vi "CODMn测量流程.vi"(11 "控制命令":u16(ring)=1 items=["启动测量"=1, "标样核查"=2, "零点核查"=3, "跨度核查"=4, "空白测试"=5, "平行样测试"=6, "加标回收"=7, "空白校准"=8, "标样校准"=9, "初始化（清洗）"=10, "停止测试"=11, "仪器重启"=12, "校时"=13, "模式设置"=14, "测量间隔设置"=15, "调试"=22, "填充管路"=30, "清洗管路"=31, "清洗反应杯"=32]) -> ()   [LabVIEW 2016, in "斯坦道CODMn新电路板.lvlib"]
panel:
  out "start":timestamp
  out "补测":bool
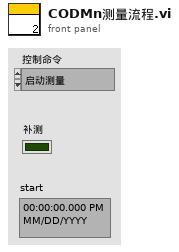
[diagram p1: front panel]
types:
  T1 = cluster{"时间标识":timestamp, "设备":string, "日志信息":string, "流程参数":string}
  T2 = cluster{"站号":u16, "量程切换":enum32{"H", "L", "AUTO"}, "控制命令":u16, "模式设置":enum16{"待机", "连续模式", "周期模式", "定点模式", "受控模式", "手动模式"}, "测量间隔":u16}
  T3 = cluster{"系统时间":timestamp, "工作状态":u16, "测量模式":enum16{"待机", "连续模式", "周期模式", "定点模式", "受控模式", "手动模式"}, "告警代码":u16, "故障代码":u16, "日志代码":u16, "软件版本":u16, "A":sgl, "B":sgl, "K":sgl, "当前滴定数":sgl, "T":sgl, "H":sgl, "id":u16, "flowid":u16, "量程":u16, "加热实时温度":sgl, "当前ORP值":sgl, "运行时间":sgl, "当前步骤剩余时间":sgl, "结束滴定数":sgl, "注射泵保温温度":sgl, "匹配滴定数X0":u16, "X^2":sgl, "X":sgl, "B 2":sgl, "光值1":sgl, "光值2":sgl, "光值3":sgl, "光值4":sgl, "光值5":sgl, "光值6":sgl, "光值7":sgl, "光值8":sgl}
  T4 = cluster{"因子编码":u32, "单位":u16, "标样参考值":sgl, "水样数据时间":timestamp, "水样实测值":sgl, "水样数据标识":string, "标样数据时间":timestamp, "标样实测值":sgl, "标样数据标识":string, "空白数据时间":timestamp, "空白实测值":sgl, "空白数据标识":string, "零点核查数据时间":timestamp, "零点核查实测值":sgl, "零点核查数据标识":string, "跨度核查数据时间":timestamp, "跨度核查实测值":sgl, "跨度核查数据标识":string, "加标回收数据时间":timestamp, "加标回收实测值":sgl, "加标回收数据标识":string, "平行样数据时间":timestamp, "平行样实测值":sgl, "平行样数据标识":string, "F0":sgl, "F1":sgl, "F2":sgl, "F3":sgl, "F4":sgl, "F5":sgl, "F6":sgl, "F7":sgl, "温度":sgl, "湿度":sgl, "X值":sgl, "fidrange":u16}
  T5 = cluster{"跨度值":dbl, "零点标准液浓度":dbl, "跨度标准液浓度":dbl, "标准液标准浓度":dbl, "零点标准液偏差":dbl, "跨度标准液偏差":dbl, "标准液标准偏差":dbl}
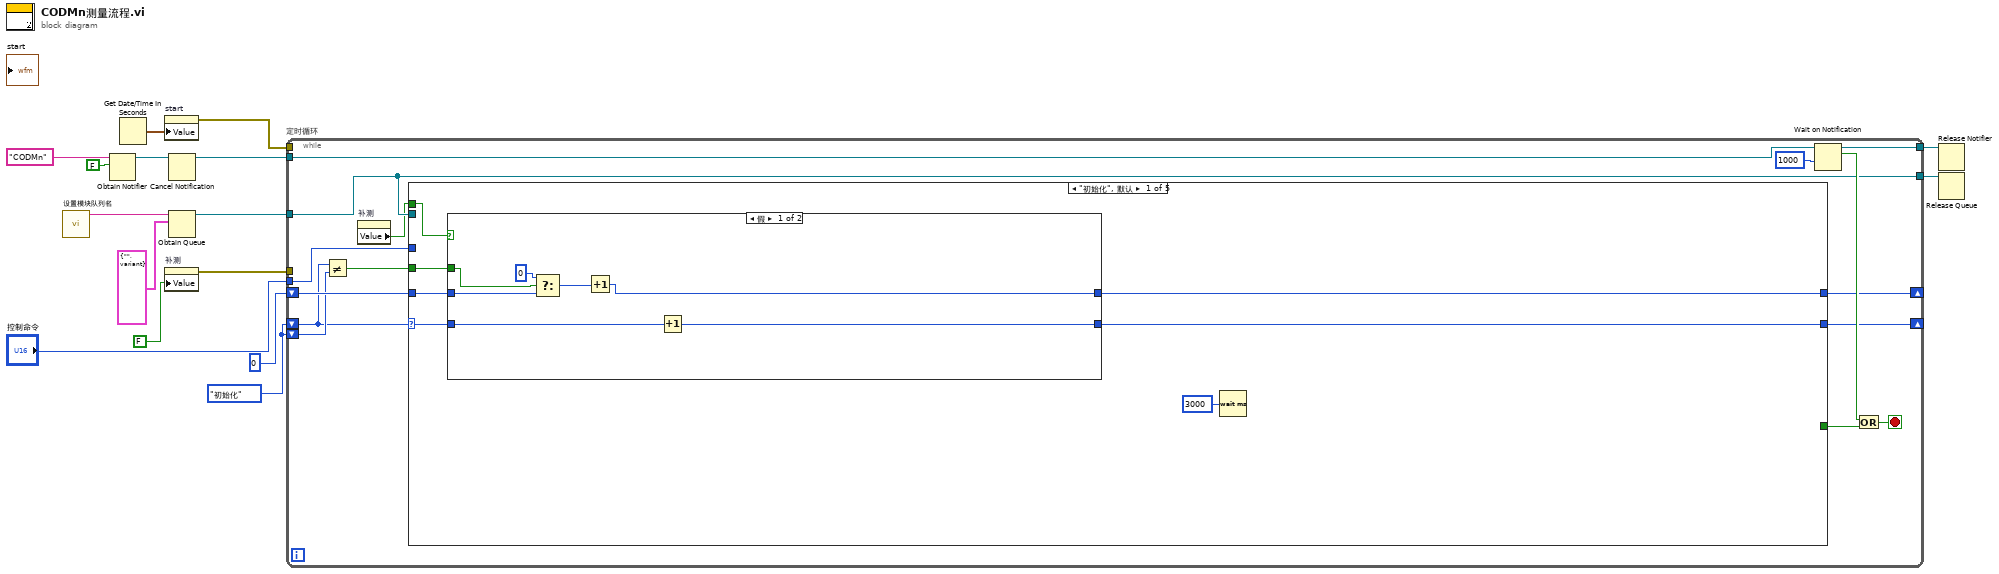
[diagram p0: block diagram]
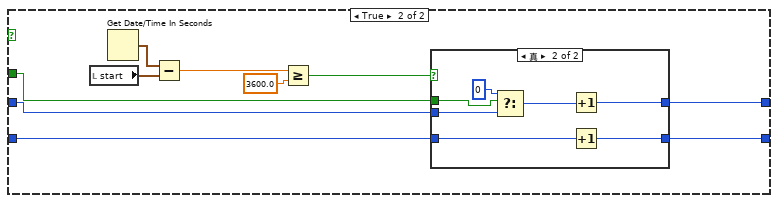
[diagram p2: hidden frame]
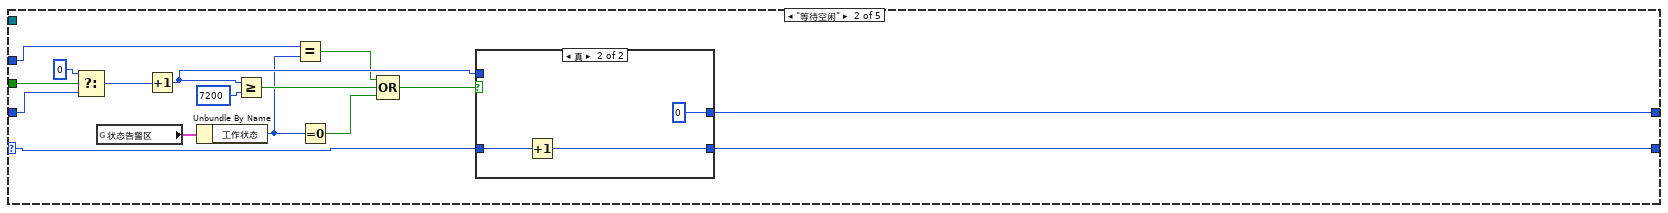
[diagram p4: hidden frame]
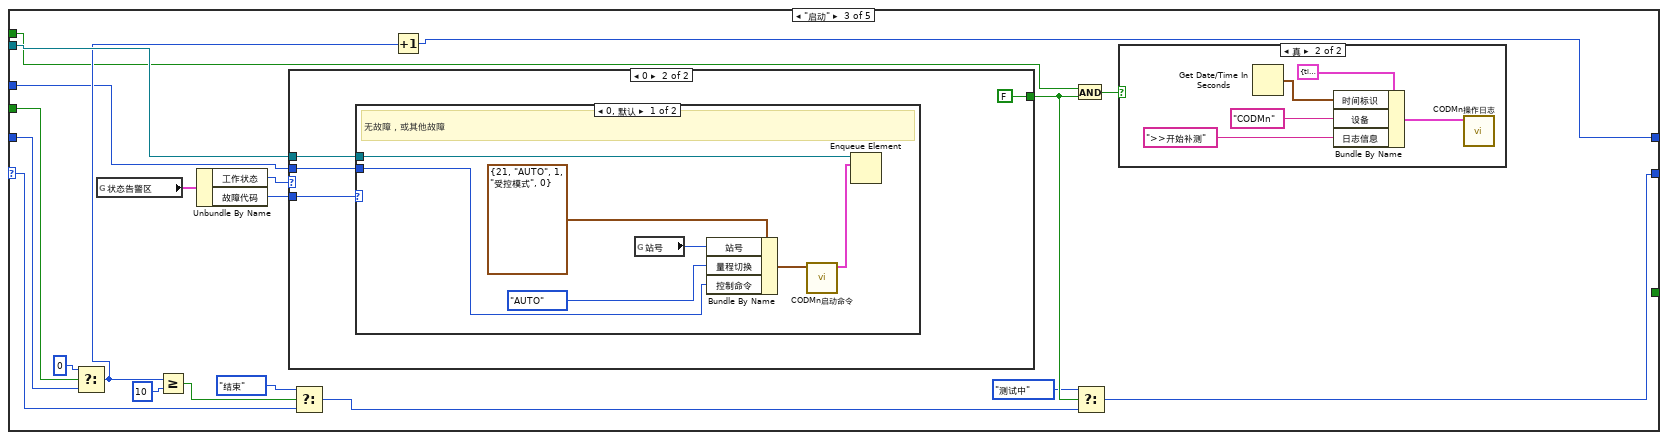
[diagram p6: hidden frame]
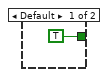
[diagram p8: hidden frame]
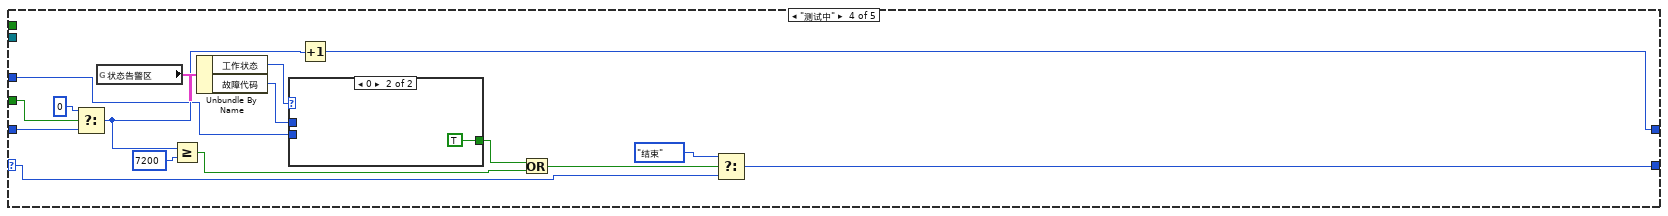
[diagram p10: hidden frame]
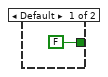
[diagram p11: hidden frame]
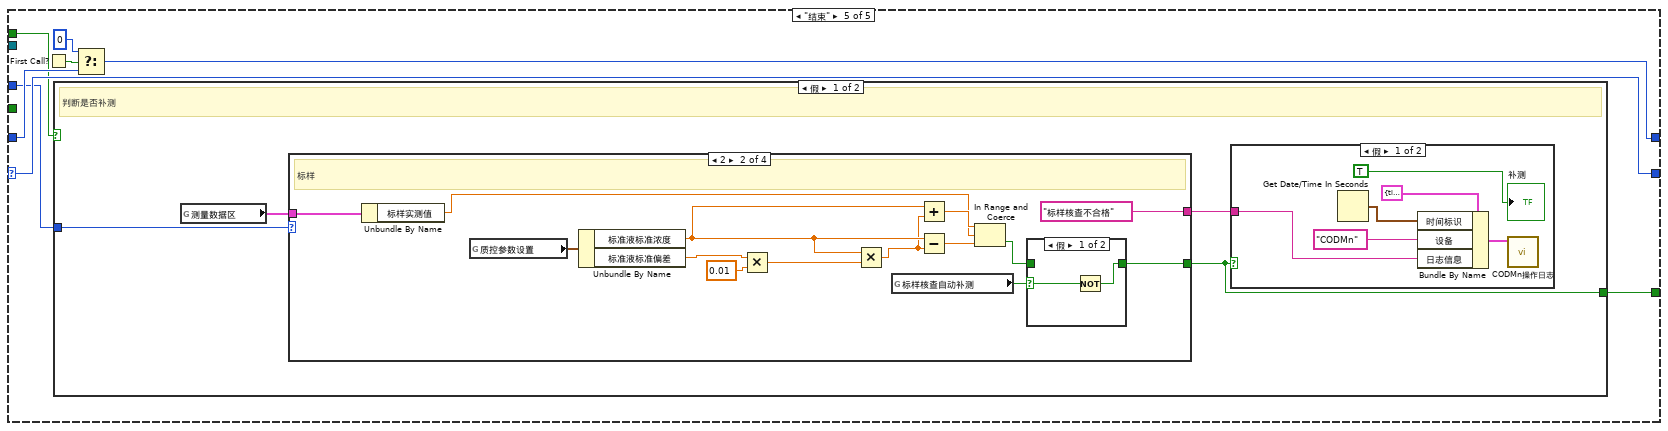
[diagram p12: hidden frame]
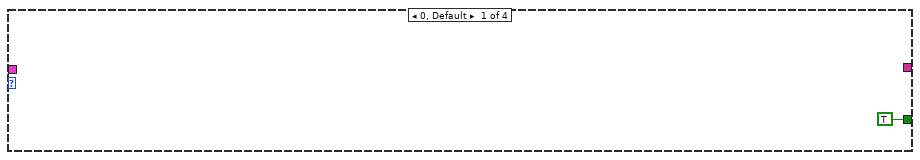
[diagram p14: hidden frame]
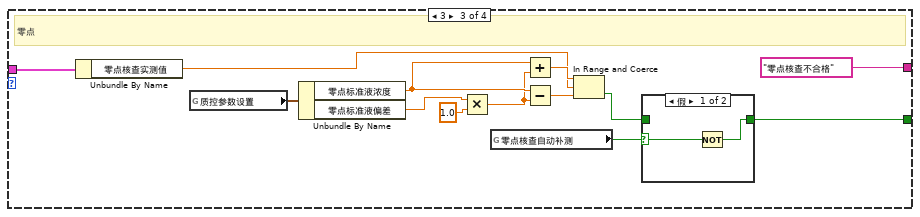
[diagram p16: hidden frame]
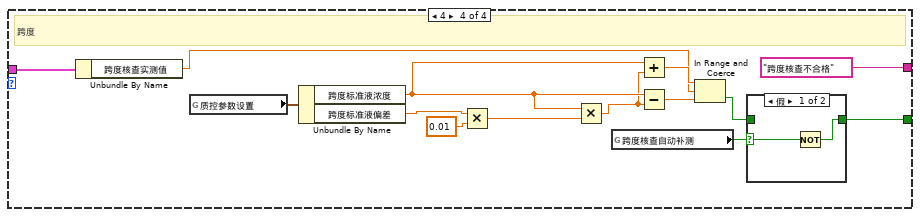
[diagram p18: hidden frame]
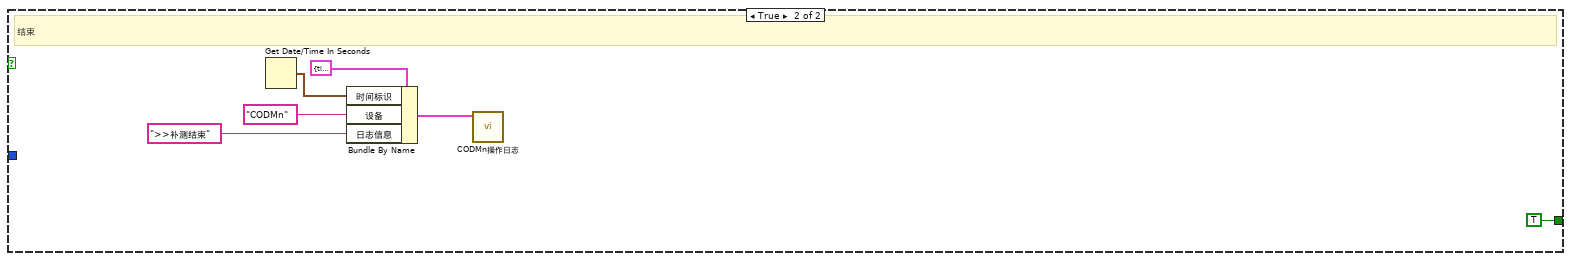
[diagram p20: hidden frame]
diagram:
  w6 = enum16{"初始化", "等待空闲", "启动", "测试中", "结束"}."初始化"
  n1 = call "设置模块队列名.vi"() -> ("Msg"=w1:string)  [unwired: 11 in]
  n2 = Obtain Notifier(name (unnamed)="CODMn" ("名称（未命名）"), notification data type=FALSE) -> (notifier out=w12:refnum<notifier>)  [unwired: 2 in, 2 out]
  n3 = Get Date/Time In Seconds() -> (seconds since 1Jan1904=w5:timestamp)
  n4 = property on="start" class="AbsTime (严格)"("Value"=w5) -> (error out=w4:errorcluster)  [unwired: 2 in, 1 out]
  n5 = property on="补测" class="Bool (严格)"("Value"=FALSE ("补测")) -> (error out=w2:errorcluster)  [unwired: 2 in, 1 out]
  n6 = Cancel Notification(0:w12) -> (8:w11:refnum<notifier>)  [unwired: 1 in, 2 out]
  n7 = Obtain Queue(name (unnamed)=w1, element data type=cluster{"命令":string, "data":variant} {"命令"="", "data"=variant}) -> (queue out=w15:refnum<queue>)  [unwired: 3 in, 2 out]
  n8 = while "定时循环" {
    tunnel: w15 -> [w21]
    tunnel: w11 -> [w31]
    tunnel: "控制命令" -> [w27]
    shift-right: [w26] -> _
    shift-left: w6 -> [w19]
    shift-right: [w24] -> _
    shift-left: 0 -> [w25]
    tunnel: [w22] -> w8
    tunnel: [w21] -> w9
    shift-left: w6 -> [w20]
    tunnel: w4 -> [_]
    tunnel: w2 -> [_]
    stop <- w28 stop-if-true
    n9 = Not Equal?(x=w19, y=w20) -> (x != y?=w18:bool)
    n10 = property on="补测" class="Bool (严格)"() -> ("Value"=w17:bool)  [unwired: 2 in, 2 out]
    n11 = case shown="\"初始化\", 默认" w19 {
      selector: w19 -> [w38 w74 w97 w130 w148]
      tunnel: w27 -> [_ w67 w95 w125 w143]
      tunnel: w21 -> [_ _ w105 _ _]
      tunnel: [w37 w69 w91 w131 w148] -> w26
      tunnel: w25 -> [w36 w77 w101 w135 w145]
      tunnel: [w35 w68 w100 w134 w144] -> w24
      tunnel: [_ _ _ _ w141] -> w23
      tunnel: w18 -> [w34 w78 w94 w124 _]
      tunnel: w17 -> [w33 _ w89 _ w142]
      frame "初始化", Default {
        n12 = case shown="假" w33 {
          tunnel: w38 -> [w41 w55]
          tunnel: [w39 w54] -> w37
          tunnel: w36 -> [w42 w53]
          tunnel: [w40 w52] -> w35
          tunnel: w34 -> [w43 w51]
          frame False {
            n13 = Select(t=0, s=w43, f=w42) -> (s? t:f=w44:i32)
            n14 = Increment(x=w44) -> (x+1=w40:i32)
            n15 = Increment(x=w41) -> (x+1=w39:enum16{"初始化", "等待空闲", "启动", "测试中", "结束"})
          }
          frame True {
            n16 = local read "start"() -> (w49:timestamp)
            n17 = Get Date/Time In Seconds() -> (seconds since 1Jan1904=w50:timestamp)
            n18 = Subtract(x=w50, y=w49) -> (x-y=w48:dbl)
            n19 = Greater Or Equal?(x=w48, y=3600.0) -> (x >= y?=w46:bool)
            n20 = case shown="真" w46 {
              tunnel: w55 -> [w57 w64]
              tunnel: [w57 w63] -> w54
              tunnel: w53 -> [w56 w62]
              tunnel: [w56 w61] -> w52
              tunnel: w51 -> [_ w60]
              frame False {
              }
              frame True {
                n21 = Select(t=0, s=w60, f=w62) -> (s? t:f=w58:i32)
                n22 = Increment(x=w58) -> (x+1=w61:i32)
                n23 = Increment(x=w64) -> (x+1=w63:enum16{"初始化", "等待空闲", "启动", "测试中", "结束"})
              }
            }
          }
        }
        n24 = Wait (ms)(milliseconds to wait=u32 3000 ("等待时间（毫秒）")) -> ()  [unwired: 1 out]
      }
      frame "等待空闲" {
        n25 = Select(t=0, s=w78, f=w77) -> (s? t:f=w79:i32)
        n26 = global read "VARCODMn全局变量.vi" "状态告警区"() -> (w75:T3)
        n27 = Increment(x=w79) -> (x+1=w70:i32)
        n28 = Unbundle By Name(w75) -> ("工作状态"=w66:u16)
        n29 = Greater Or Equal?(x=w70, y=7200) -> (x >= y?=w73:bool)
        n30 = Equal?(x=w67, y=w66) -> (x = y?=w65:bool)
        n31 = Equal To 0?(x=w66) -> (x = 0?=w72:bool)
        n32 = Compound Arithmetic op=OR ("复合运算")(w65, w73, w72) -> (w71:bool)
        n33 = case shown="真" w71 {
          tunnel: w74 -> [w81 w85]
          tunnel: w70 -> [w82 _]
          tunnel: [w81 w84] -> w69
          tunnel: [w82 0] -> w68
          frame False {
          }
          frame True {
            n34 = Increment(x=w85) -> (x+1=w84:enum16{"初始化", "等待空闲", "启动", "测试中", "结束"})
          }
        }
      }
      frame "启动" {
        n35 = Select(t=0, s=w94, f=w101) -> (s? t:f=w99:i32)
        n36 = global read "VARCODMn全局变量.vi" "状态告警区"() -> (w104:T3)
        n37 = Greater Or Equal?(x=w99, y=10) -> (x >= y?=w92:bool)
        n38 = Unbundle By Name(w104) -> ("工作状态"=w103:u16, "故障代码"=w96:u16)
        n39 = case shown="0" w103 {
          tunnel: w95 -> [_ w114]
          tunnel: w105 -> [_ w115]
          tunnel: [TRUE FALSE] -> w90
          tunnel: w96 -> [_ w113]
          frame Default {
          }
          frame 0 {
            n40 = case shown="0, 默认" w113 {
              tunnel: w115 -> [w121 _]
              tunnel: w114 -> [w120 _]
              frame 0, Default {
                # "无故障，或其他故障"
                n41 = global read "CODMn断电保存全局变量.vi" "站号"() -> (w119:u16)
                n42 = Bundle By Name(cluster=T2 {"站号"=21, "量程切换"=enum."AUTO", "控制命令"=1, "模式设置"=enum."受控模式", "测量间隔"=0} ("参数"), "站号"=w119, "量程切换"=enum32{"H", "L", "AUTO"}."AUTO", "控制命令"=w120) -> (w116:T2)
                n43 = call "CODMn启动命令.vi"("参数"=w116) -> ("启动命令"=w122:cluster{"命令":string, "data":variant})  [unwired: 10 in]
                n44 = Enqueue Element(queue=w121, element=w122) -> ()  [unwired: 2 in, 3 out]
              }
              frame 2 {
                # "加热故障"
              }
            }
          }
        }
        n45 = Select(t=enum16{"初始化", "等待空闲", "启动", "测试中", "结束"}."结束", s=w92, f=w97) -> (s? t:f=w93:enum16{"初始化", "等待空闲", "启动", "测试中", "结束"})
        n46 = Increment(x=w99) -> (x+1=w100:i32)
        n47 = And(x=w89, y=w90) -> (x .and. y?=w88:bool)
        n48 = Select(t=enum16{"初始化", "等待空闲", "启动", "测试中", "结束"}."测试中", s=w90, f=w93) -> (s? t:f=w91:enum16{"初始化", "等待空闲", "启动", "测试中", "结束"})
        n49 = case shown="真" w88 {
          frame False {
          }
          frame True {
            n50 = Get Date/Time In Seconds() -> (seconds since 1Jan1904=w108:timestamp)
            n51 = Bundle By Name(cluster=T1 {"时间标识"=timestamp(0 s since 1904-01-01), "设备"="", "日志信息"="", "流程参数"=""} ("data in"), "时间标识"=w108, "设备"="CODMn", "日志信息"=">>开始补测") -> (w110:T1)
            n52 = call "CODMn操作日志.vi"("data in"=w110) -> ()  [unwired: 11 in]
          }
        }
      }
      frame "测试中" {
        n53 = Select(t=0, s=w124, f=w135) -> (s? t:f=w133:i32)
        n54 = global read "VARCODMn全局变量.vi" "状态告警区"() -> (w138:T3)
        n55 = Greater Or Equal?(x=w133, y=7200) -> (x >= y?=w129:bool)
        n56 = Unbundle By Name(w138) -> ("工作状态"=w137:u16, "故障代码"=w126:u16)
        n57 = case shown="0" w137 {
          tunnel: w125 -> [_ _]
          tunnel: [FALSE TRUE] -> w127
          tunnel: w126 -> [_ _]
          frame Default {
          }
          frame 0 {
          }
        }
        n58 = Increment(x=w133) -> (x+1=w134:i32)
        n59 = Or(x=w127, y=w129) -> (x .or. y?=w128:bool)
        n60 = Select(t=enum16{"初始化", "等待空闲", "启动", "测试中", "结束"}."结束", s=w128, f=w130) -> (s? t:f=w131:enum16{"初始化", "等待空闲", "启动", "测试中", "结束"})
      }
      frame "结束" {
        n61 = First Call?() -> (First Call?: T/F=w147:bool)
        n62 = case shown="假" w142 {
          tunnel: w143 -> [w152 _]
          tunnel: [w149 TRUE] -> w141
          frame False {
            # "判断是否补测"
            n63 = global read "VARCODMn全局变量.vi" "测量数据区"() -> (w151:T4)
            n64 = case shown="2" w152 {
              tunnel: w151 -> [_ w173 w179 w198]
              tunnel: [TRUE w164 w178 w197] -> w149
              tunnel: [_ "标样核查不合格" ("日志信息") "零点核查不合格" ("日志信息") "跨度核查不合格" ("日志信息")] -> w150
              frame 0, Default {
              }
              frame 2 {
                # "标样"
                n65 = Unbundle By Name(w173) -> ("标样实测值"=w165:sgl)
                n66 = global read "CODMn断电保存全局变量.vi" "质控参数设置"() -> (w166:T5)
                n67 = Unbundle By Name(w166) -> ("标准液标准浓度"=w161:dbl, "标准液标准偏差"=w168:dbl)
                n68 = Multiply(x=w168, y=0.01) -> (x*y=w162:dbl)
                n69 = Multiply(x=w161, y=w162) -> (x*y=w160:dbl)
                n70 = global read "CODMn断电保存全局变量.vi" "标样核查自动补测"() -> (w171:bool)
                n71 = Add(x=w161, y=w160) -> (x+y=w169:dbl)
                n72 = Subtract(x=w161, y=w160) -> (x-y=w170:dbl)
                n73 = In Range and Coerce(upper limit=w169, x=w165, lower limit=w170) -> (In Range?=w172:bool)  [unwired: 1 out]
                n74 = case shown="假" w171 {
                  selector: w171 -> [w175 _]
                  tunnel: w172 -> [_ w176]
                  tunnel: [w174 w176] -> w164
                  frame False {
                    n75 = Not(x=w175) -> (.not. x?=w174:bool)
                  }
                  frame True {
                  }
                }
              }
              frame 3 {
                # "零点"
                n76 = Unbundle By Name(w179) -> ("零点核查实测值"=w180:sgl)
                n77 = global read "CODMn断电保存全局变量.vi" "质控参数设置"() -> (w181:T5)
                n78 = Unbundle By Name(w181) -> ("零点标准液浓度"=w184:dbl, "零点标准液偏差"=w185:dbl)
                n79 = Multiply(x=w185, y=1.0) -> (x*y=w183:dbl)
                n80 = global read "CODMn断电保存全局变量.vi" "零点核查自动补测"() -> (w188:bool)
                n81 = Add(x=w184, y=w183) -> (x+y=w186:dbl)
                n82 = Subtract(x=w184, y=w183) -> (x-y=w187:dbl)
                n83 = In Range and Coerce(upper limit=w186, x=w180, lower limit=w187) -> (In Range?=w189:bool)  [unwired: 1 out]
                n84 = case shown="假" w188 {
                  selector: w188 -> [w191 _]
                  tunnel: w189 -> [_ w192]
                  tunnel: [w190 w192] -> w178
                  frame False {
                    n85 = Not(x=w191) -> (.not. x?=w190:bool)
                  }
                  frame True {
                  }
                }
              }
              frame 4 {
                # "跨度"
                n86 = Unbundle By Name(w198) -> ("跨度核查实测值"=w199:sgl)
                n87 = global read "CODMn断电保存全局变量.vi" "质控参数设置"() -> (w200:T5)
                n88 = Unbundle By Name(w200) -> ("跨度标准液浓度"=w194:dbl, "跨度标准液偏差"=w202:dbl)
                n89 = Multiply(x=w202, y=0.01) -> (x*y=w195:dbl)
                n90 = Multiply(x=w194, y=w195) -> (x*y=w193:dbl)
                n91 = global read "CODMn断电保存全局变量.vi" "跨度核查自动补测"() -> (w205:bool)
                n92 = Add(x=w194, y=w193) -> (x+y=w203:dbl)
                n93 = Subtract(x=w194, y=w193) -> (x-y=w204:dbl)
                n94 = In Range and Coerce(upper limit=w203, x=w199, lower limit=w204) -> (In Range?=w206:bool)  [unwired: 1 out]
                n95 = case shown="假" w205 {
                  selector: w205 -> [w208 _]
                  tunnel: w206 -> [_ w209]
                  tunnel: [w207 w209] -> w197
                  frame False {
                    n96 = Not(x=w208) -> (.not. x?=w207:bool)
                  }
                  frame True {
                  }
                }
              }
            }
            n97 = case shown="假" w149 {
              tunnel: w150 -> [w154 _]
              frame False {
                n98 = Get Date/Time In Seconds() -> (seconds since 1Jan1904=w156:timestamp)
                n99 = Bundle By Name(cluster=T1 {"时间标识"=timestamp(0 s since 1904-01-01), "设备"="", "日志信息"="", "流程参数"=""} ("data in"), "时间标识"=w156, "设备"="CODMn", "日志信息"=w154) -> (w155:T1)
                n100 = call "CODMn操作日志.vi"("data in"=w155) -> ()  [unwired: 11 in]
                "补测" <- TRUE ("补测")
              }
              frame True {
              }
            }
          }
          frame True {
            # "结束"
            n101 = Get Date/Time In Seconds() -> (seconds since 1Jan1904=w212:timestamp)
            n102 = Bundle By Name(cluster=T1 {"时间标识"=timestamp(0 s since 1904-01-01), "设备"="", "日志信息"="", "流程参数"=""} ("data in"), "时间标识"=w212, "设备"="CODMn", "日志信息"=">>补测结束") -> (w214:T1)
            n103 = call "CODMn操作日志.vi"("data in"=w214) -> ()  [unwired: 11 in]
          }
        }
        n104 = Select(t=0, s=w147, f=w145) -> (s? t:f=w144:i32)
      }
    }
    n105 = Wait on Notification(notifier=w31, timeout in ms (-1)=1000 ("超时毫秒(-1)")) -> (notifier out=w22:refnum<notifier>, notification=w29:bool)  [unwired: 2 in, 2 out]
    n106 = Or(x=w29, y=w23) -> (x .or. y?=w28:bool)
  }
  n107 = Release Notifier(notifier=w8) -> ()  [unwired: 2 in, 3 out]
  n108 = Release Queue(queue=w9) -> ()  [unwired: 2 in, 3 out]
